vi "TelnetTest.vi"() -> ()   [LabVIEW 2018]
uses:
  Telnet V2.lvclass
panel:
  in  "Input":string
  in  "stop":bool
  out "Output":string
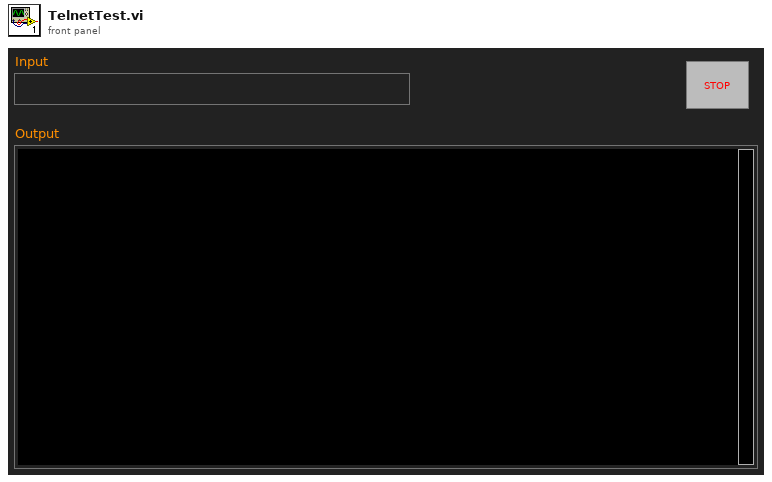
[diagram p1: front panel]
types:
  T1 = typedef "eventvkey.ctl" = enum16{"ASCII", "Enter", "Return", "Shift", "Ctrl", "Alt", "Cmd", "Opt", "Caps", "NumLock", "Clear", "Break", "Up", "Down", "Left", "Right", "Insert", "Delete", "Home", "End", "PageUp", "PageDown", "Escape", "Help", "Pause", "ScrollLock", "F1", "F2", "F3", "F4", "F5", "F6", "F7", "F8", "F9", "F10", "F11", "F12", "F13", "F14", "F15", "F16", "F17", "F18", "F19", "F20", "F21", "F22", "F23", "F24", "Play", "VolumeUp", "VolumeDown", "Mute", "Two Byte Char"}
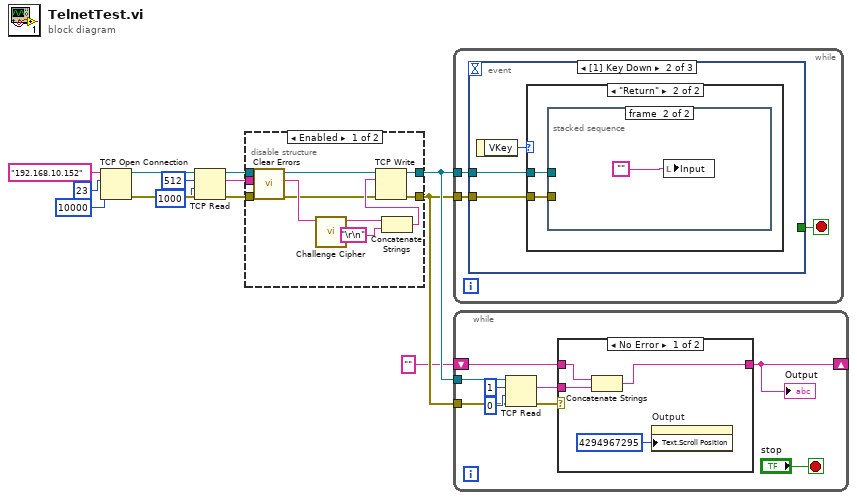
[diagram p0: block diagram]
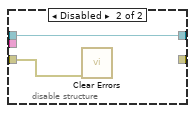
[diagram p2: hidden frame]
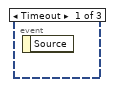
[diagram p3: hidden frame]
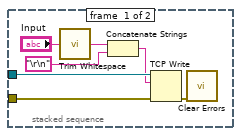
[diagram p5: hidden frame]
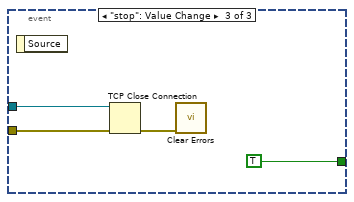
[diagram p6: hidden frame]
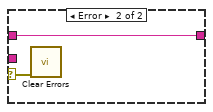
[diagram p7: hidden frame]
diagram:
  n1 = TCP Open Connection(address="192.168.10.152", remote port or service name=u16 23, timeout ms (60000)=10000) -> (connection ID=w12:refnum<k5>, error out=w13:errorcluster)  [unwired: 2 in]
  n2 = TCP Read(connection ID=w12, bytes to read=512, error in (no error)=w13, 9:1000 ("timeout ms (25000)")) -> (connection ID out=w5:refnum<k5>, data out=w4:string, error out=w6:errorcluster)  [unwired: 1 in]
  n3 = disable-structure shown="Enabled" {
    disable-tunnel: w6 -> [w22 w23]
    disable-tunnel: w5 -> [w21 w24]
    disable-tunnel: w4 -> [w17 _]
    disable-tunnel: [w15 w24] -> w3
    disable-tunnel: [w14 _] -> w2
    frame Enabled {
      n4 = call <vilib>:"Clear Errors.vi"("error in (no error)"=w22) -> ("error out"=w16:errorcluster)  [unwired: 5 in, 1 out]
      n5 = call "Challenge Cipher.vi"("Message In"=w17) -> ("Response"=w20:string)  [unwired: 10 in]
      n6 = Concatenate Strings(w20, "\r\n") -> (w18:string)
      n7 = TCP Write(connection ID=w21, data in=w18, error in (no error)=w16) -> (connection ID out=w15:refnum<k5>, error out=w14:errorcluster)  [unwired: 1 in, 1 out]
    }
    frame Disabled {
      n8 = call <vilib>:"Clear Errors.vi"("error in (no error)"=w23) -> ()  [unwired: 5 in, 2 out]
    }
  }
  n9 = while {
    tunnel: w3 -> [w27]
    tunnel: w2 -> [w26]
    stop <- w25 stop-if-true
    n10 = event shown="[1] Key Down" {
      selector: _ -> [_ _ _]
      dyn-events: _ -> [_ _ _]
      timeout: _ -> [_ _ _]
      tunnel: w27 -> [_ w29 w43]
      tunnel: w26 -> [_ w28 w42]
      tunnel: [_ _ TRUE] -> w25
      event Timeout {
        n11 = event-data() -> ()  [unwired: 1 in, 1 out]
      }
      event Key Down {
        n12 = event-data() -> ("VKey"=w30:T1)  [unwired: 1 in]
        n13 = case shown="\"Return\"" w30 {
          tunnel: w29 -> [_ w32]
          tunnel: w28 -> [_ w31]
          frame Default {
          }
          frame "Return" {
            n14 = stacked-sequence {
              tunnel: w32 -> [w39 _]
              tunnel: w31 -> [w38 _]
              frame #0 {
                n15 = call <vilib>:"Trim Whitespace.vi"("string"="Input") -> ("trimmed string"=w33:string)  [unwired: 1 in]
                n16 = Concatenate Strings(w33, "\r\n") -> (w34:string)
                n17 = TCP Write(connection ID=w39, data in=w34, error in (no error)=w38) -> (error out=w37:errorcluster)  [unwired: 1 in, 2 out]
                n18 = call <vilib>:"Clear Errors.vi"("error in (no error)"=w37) -> ()  [unwired: 5 in, 2 out]
              }
              frame #1 {
                n19 = local write "Input"("") -> ()
              }
            }
          }
        }
      }
      event "stop": Value Change {
        n20 = event-data() -> ()  [unwired: 1 in, 1 out]
        n21 = TCP Close Connection(connection ID=w43, error in (no error)=w42) -> (error out=w41:errorcluster)  [unwired: 1 in, 1 out]
        n22 = call <vilib>:"Clear Errors.vi"("error in (no error)"=w41) -> ()  [unwired: 5 in, 2 out]
      }
    }
  }
  n23 = while {
    tunnel: w3 -> [w51]
    tunnel: w2 -> [w50]
    shift-right: [w45] -> _
    shift-left: "" -> [w47]
    stop <- "stop" stop-if-true
    n24 = TCP Read(connection ID=w51, bytes to read=1, error in (no error)=w50, 9:0 ("timeout ms (25000)")) -> (data out=w48:string, error out=w49:errorcluster)  [unwired: 1 in, 1 out]
    n25 = case shown="No Error" w49 {
      selector: w49 -> [_ w58]
      tunnel: w48 -> [w57 _]
      tunnel: [w55 w59] -> w45
      tunnel: w47 -> [w56 w59]
      frame No Error {
        n26 = Concatenate Strings(w56, w57) -> (w55:string)
        n27 = property on="Output" class="Str"("Text.Scroll Position"=u32 4294967295) -> ()  [unwired: 2 in, 2 out]
      }
      frame Error {
        n28 = call <vilib>:"Clear Errors.vi"("error in (no error)"=w58) -> ()  [unwired: 5 in, 2 out]
      }
    }
    "Output" <- w45
  }
